vi "sensor cmd sample get.vi"(9 "buff_length":i32, 10 "dest_buffer":string, 11 "device_handle":u32) -> (1 "function return":i32, 2 "dest_buffer out":string, 3 "device_handle out":u32)   [LabVIEW 2019, in "apdm.lvlib"]
doc: "APDM_EXPORT int apdm_sensor_cmd_sample_get(apdm_device_handle_t device_handle, uint8_t *dest_buffer, const int buff_length);"
uses:
  apdm.lvlib
  Lee Lab/CP FES Walking 2018/Code/Working/LabVIEW/apdm.dll
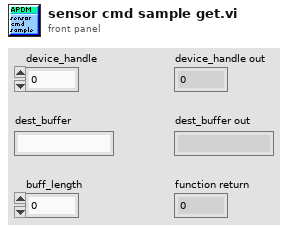
[diagram p1: front panel]
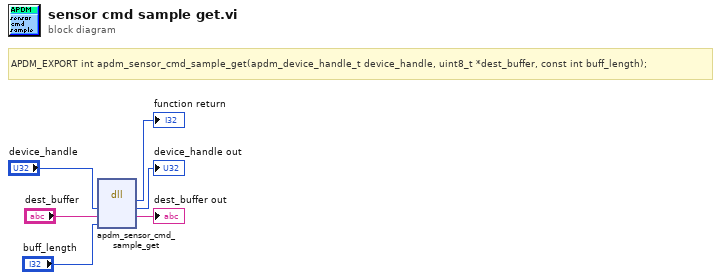
[diagram p0: block diagram]
diagram:
  # "APDM_EXPORT int apdm_sensor_cmd_sample_get(apdm_device_handle_t device_handle, uint8_t *dest_buffer, const int buff_length);"
  n1 = dll-call lib="C:/Users/jfalesi/Dropbox/Lee Lab/CP FES Walking 2018/Code/Working/LabVIEW/apdm.*" fn="apdm_sensor_cmd_sample_get"("device_handle"="device_handle", "dest_buffer"="dest_buffer", "buff_length"="buff_length") -> (→"function return":i32, "device_handle"=→"device_handle out":u32, "dest_buffer"=→"dest_buffer out":string)  [unwired: 4 in, 2 out]
